vi "Reorientate_student.vi"(9 "Roll":dbl, 10 "Pitch":dbl, 11 "Vector (x, y, z)":dbl[](array[numeric])) -> (1 "Rz":dbl, 2 "Ry":dbl, 3 "Rx":dbl)   [LabVIEW 2014]
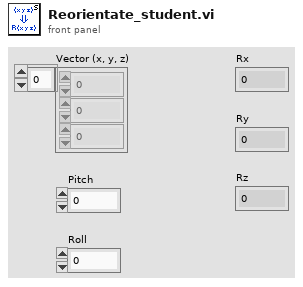
[diagram p1: front panel]
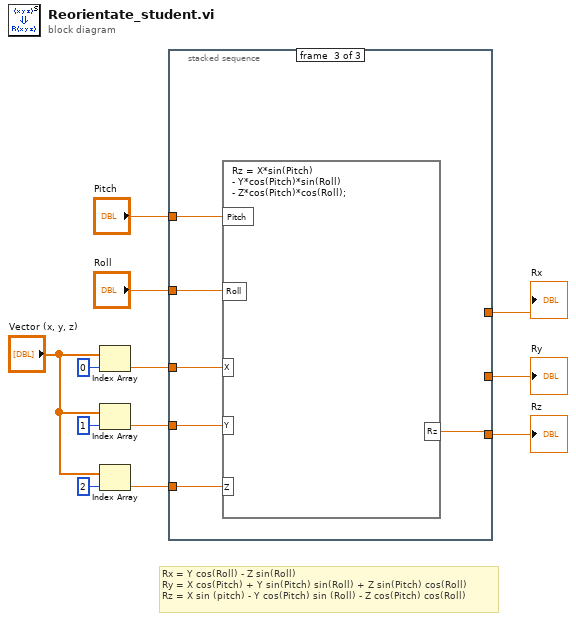
[diagram p0: block diagram]
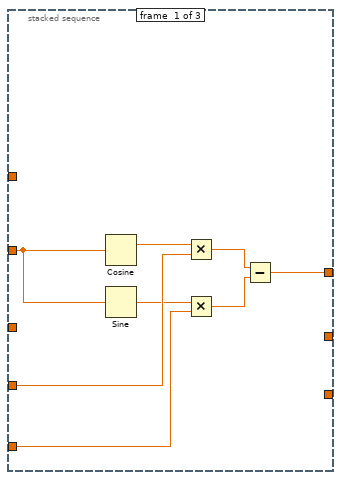
[diagram p2: hidden frame]
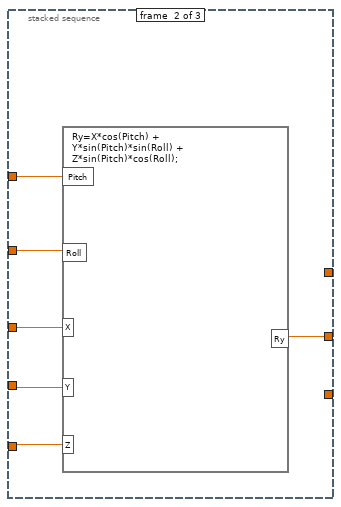
[diagram p3: hidden frame]
diagram:
  # "Rx = Y cos(Roll) - Z sin(Roll)\nRy = X cos(Pitch) + Y sin(Pitch) sin(Roll) + Z sin(Pitch) cos(Roll)\nRz = X sin (pitch) - Y cos(Pitch) sin (Roll) - Z cos(Pitch) cos(Roll)"
  n1 = Index Array(array="Vector (x, y, z)", index=0) -> (element=w9:dbl)
  n2 = Index Array(array="Vector (x, y, z)", index=1) -> (element=w5:dbl)
  n3 = Index Array(array="Vector (x, y, z)", index=2) -> (element=w6:dbl)
  n4 = stacked-sequence {
    tunnel: "Roll" -> [w18 w25 w31]
    tunnel: w5 -> [w20 w22 w29]
    tunnel: w6 -> [w17 w24 w28]
    tunnel: w9 -> [_ w23 w30]
    tunnel: "Pitch" -> [_ w26 w32]
    tunnel: [w14 _ _] -> w3
    tunnel: [_ w21 _] -> w2
    tunnel: [_ _ w27] -> w1
    frame #0 {
      n5 = Cosine(x=w18) -> (cos(x)=w19:dbl)
      n6 = Sine(x=w18) -> (sin(x)=w15:dbl)
      n7 = Multiply(x=w19, y=w20) -> (x*y=w16:dbl)
      n8 = Multiply(x=w15, y=w17) -> (x*y=w13:dbl)
      n9 = Subtract(x=w16, y=w13) -> (x-y=w14:dbl)
    }
    frame #1 {
      n10 = formula code="Ry=X*cos(Pitch) + \nY*sin(Pitch)*sin(Roll) + \nZ*sin(Pitch)*cos(Roll);"("Pitch"=w26, "Roll"=w25, "Z"=w24, "Y"=w22, "X"=w23) -> ("Ry"=w21:dbl)
    }
    frame #2 {
      n11 = formula code="Rz = X*sin(Pitch)\n- Y*cos(Pitch)*sin(Roll)\n- Z*cos(Pitch)*cos(Roll);"("Pitch"=w32, "Roll"=w31, "X"=w30, "Y"=w29, "Z"=w28) -> ("Rz"=w27:dbl)
    }
  }
  "Ry" <- w2
  "Rx" <- w3
  "Rz" <- w1
